vi "setAsServer.vi"(10 "server":bool, 11 "Connection in":refnum<class "Connection.lvclass">) -> (3 "Connection out":refnum<class "Connection.lvclass">)   [LabVIEW 2013, in "Connection_GOSPL.lvlib" / "Connection.lvclass"]
uses:
  Connection.lvclass
  Connection.lvclass/Connection.ctl
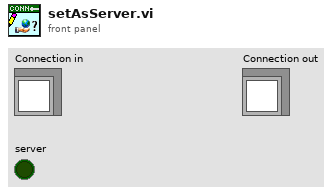
[diagram p1: front panel]
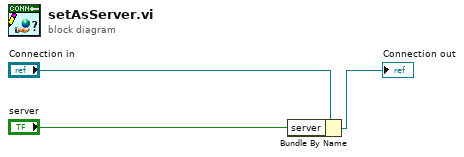
[diagram p0: block diagram]
diagram:
  n1 = Bundle By Name(cluster="Connection in", "server"="server") -> (→"Connection out":refnum<class "Connection.lvclass">)
